vi "calcTime.vi"(8 "error in (no error)":errorcluster, 10 "Steering Angle":dbl) -> (0 "error (out)":errorcluster, 1 "Active Actuator Time":dbl, 2 "Positive Angle?":bool)   [LabVIEW 2015]
doc: "Convert the steering angle to the actuator active time and whether or not the actuator should extend or retract."
uses:
  <vilib>/express/express arith-compare/Formula/XNode/ExpressFormulaBlockNode.xnode
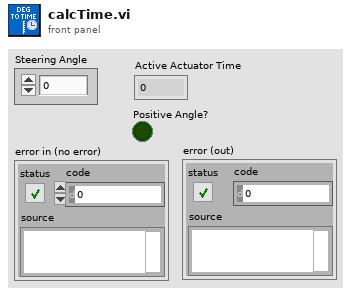
[diagram p1: front panel]
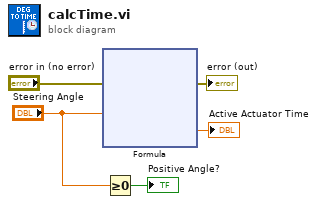
[diagram p0: block diagram]
diagram:
  n1 = xnode "Formula"("Angle"="Steering Angle", "error in (no error)"="error in (no error)") -> ("Result"=→"Active Actuator Time":dbl, "error out"=→"error (out)":errorcluster)
  n2 = Greater Or Equal To 0?(x="Steering Angle") -> (x >= 0?=→"Positive Angle?":bool)
